vi "Read and Return AI Task.vi"(0 "AI Task In":refnum<k21>[](array[refnum])=["", ""], 1 "AI Block Size In":i32=5000, 2 "AI Buffer Size (s) In":i32=10, 3 "AI Rate In":dbl=10000.0 format="%.2f") -> (5 "Input Signal Out":dbl[][](graph), 6 "Backlog Out":u8(slide) scale=0.0..100.0)   [LabVIEW 2013, in "Lock-In Variable Channels_2.lvclass"]
uses:
  Lock-In Variable Channels_2.lvclass
panel:
  out "Signal Out":dbl[][](array[numeric])
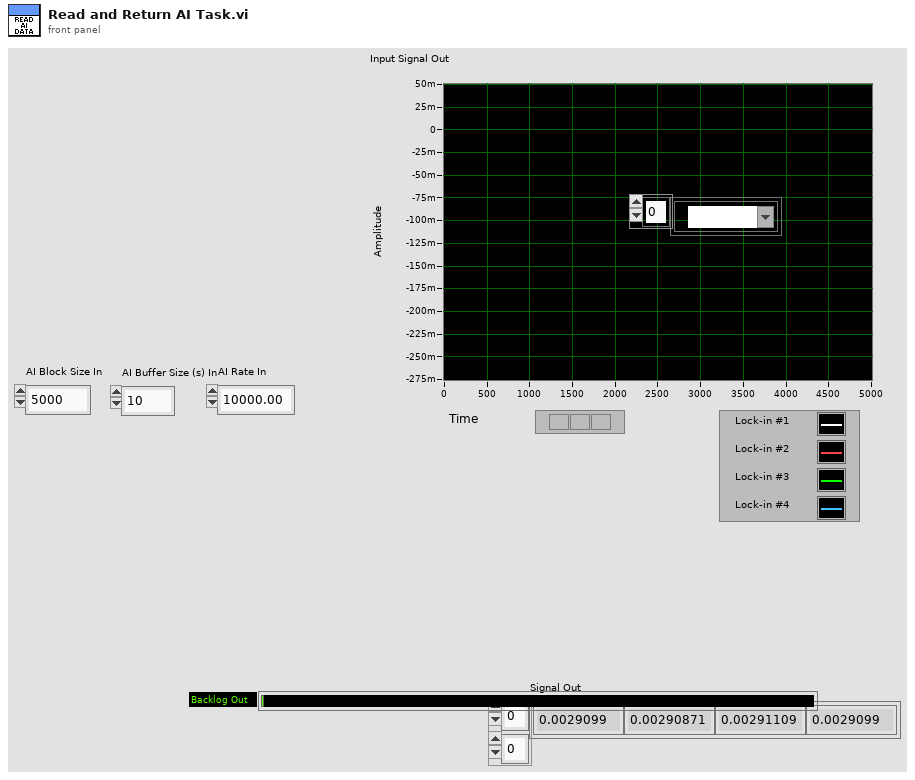
[diagram p1: front panel]
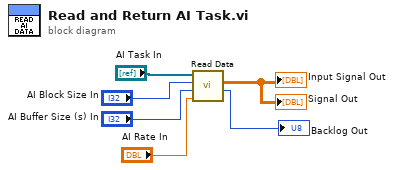
[diagram p0: block diagram]
diagram:
  n1 = call "Read Data.vi"("AI Rate"="AI Rate In", "AI Buffer Size (s)"="AI Buffer Size (s) In", "AI Block Size"="AI Block Size In", "AI task"="AI Task In") -> ("Backlog"=→"Backlog Out":u8, "Input Signals"=→"Signal Out" →"Input Signal Out":dbl[][])  [unwired: 6 in]
